vi "Test Add.vi"(8 "error in (no error)":errorcluster, 10 "Test Record":T1, 11 "Connection Refnum":T2) -> (0 "error out":errorcluster, 2 "New Test Record":T1, 3 "Connection Refnum":T2)   [LabVIEW 2011]
uses:
  Test Record.ctl
  Summitek EXT/ODBC/SQL Controls/Connection Refnum.ctl
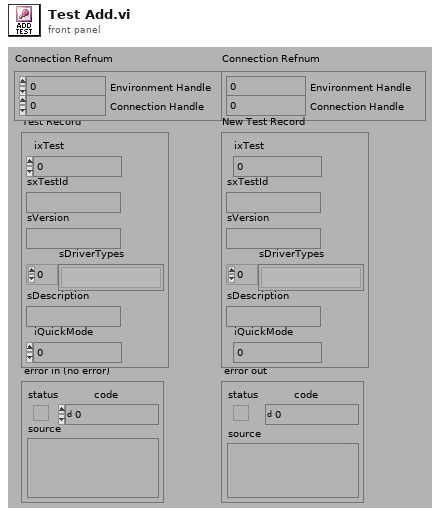
[diagram p1: front panel]
types:
  T1 = typedef "Test Record.ctl" = cluster{"ixTest":i32, "sxTestId":string, "sVersion":string, "sDriverTypes":string[], "sDescription":string, "iQuickMode":i32}
  T2 = typedef "Connection Refnum.ctl" = cluster{"Environment Handle":i32, "Connection Handle":i32}
  T3 = typedef "Statement Refnum.ctl" = cluster{"Statement Handle":i32, "Parameter Number":u16}
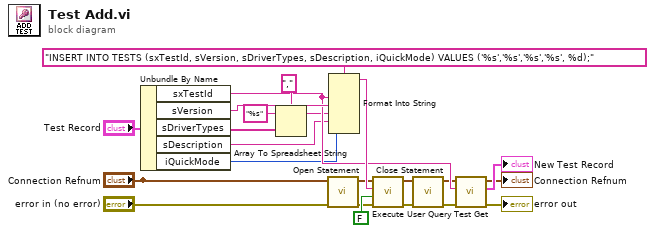
[diagram p0: block diagram]
diagram:
  n1 = Unbundle By Name("Test Record") -> ("sxTestId"=w8:string, "sVersion"=w12:string, "sDriverTypes"=w11:string[], "sDescription"=w3:string, "iQuickMode"=w7:i32)
  n2 = Array To Spreadsheet String(delimiter (Tab)=",", array=w11, 3:"%s" ("format string")) -> (spreadsheet string=w4:string)
  n3 = call "Open Statement.vi"("error in (no error)"="error in (no error)", "Connection Refnum"="Connection Refnum") -> ("error out"=w17:errorcluster, "Statement Refnum"=w16:T3)  [unwired: 4 out]
  n4 = Format Into String(format string="INSERT INTO TESTS (sxTestId, sVersion, sDriverTypes, sDescription, iQuickMode) VALUES ('%s','%s','%s','%s', %d);" ("User Query"), w8, w12, w4, w3, w7) -> (resulting string=w21:string)  [unwired: 2 in, 1 out]
  n5 = call "Execute User Query.vi"("error in (no error)"=w17, "Return Data? (f)"=FALSE, "User Query"=w21, "Statement Refnum"=w16) -> ("error out"=w18:errorcluster, "Statement Refnum"=w19:T3)  [unwired: 2 out]
  n6 = call "Close Statement.vi"("error in (no error)"=w18, "Statement Refnum"=w19) -> ("error out"=w14:errorcluster)  [unwired: 5 out]
  n7 = call "Test Get.vi"("error in (no error)"=w14, "Test_ID"=w8, "Connection Refnum"="Connection Refnum") -> ("error out"=→"error out":errorcluster, "Test Record"=→"New Test Record":T1, "Connection Refnum"=→"Connection Refnum":T2)  [unwired: 6 out]
